vi "ke37xx Configure Filter.vi"(0 "VISA Resource Name":refnum<visa-resource-name>, 5 "Enabled (False)":bool, 7 "Filter Count (1)":u8=1 min=1 max=100, 9 "Filter Type (0: Repeating Average)":enum16{"Repeating Average", "Moving Average"}(ring), 11 "error in (no error)":errorcluster, 12 "Window (0.1)":dbl=0.1 min=0.0 max=10.0) -> (4 "VISA Resource Name Out":refnum<visa-resource-name>, 15 "error out":errorcluster)   [LabVIEW 2009, in "Keithley 3700 Series.lvlib"]
doc: "This VI allows you to configure the measurement filter."
uses:
  <instrlib>/Keithley 3706/Keithley 3700 Series.lvlib
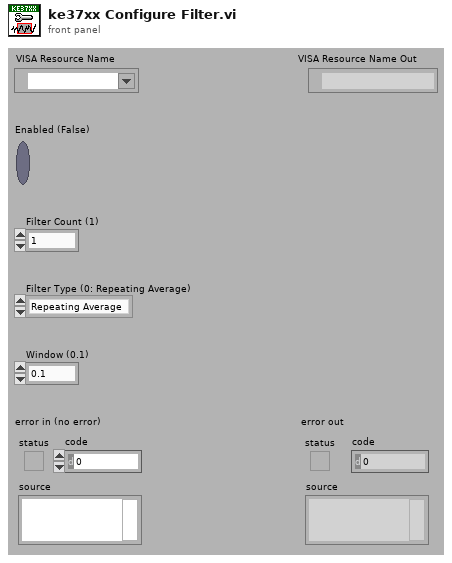
[diagram p1: front panel]
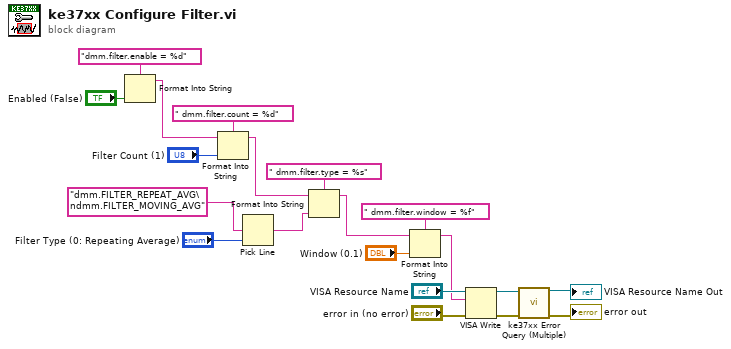
[diagram p0: block diagram]
diagram:
  n1 = Format Into String(format string="dmm.filter.enable = %d", "Enabled (False)") -> (resulting string=w8:string)  [unwired: 2 in, 1 out]
  n2 = Format Into String(format string=" dmm.filter.count = %d", initial string=w8, "Filter Count (1)") -> (resulting string=w7:string)  [unwired: 1 in, 1 out]
  n3 = Pick Line(multi-line string="dmm.FILTER_REPEAT_AVG\ndmm.FILTER_MOVING_AVG", line index="Filter Type (0: Repeating Average)") -> (output string=w2:string)  [unwired: 1 out]
  n4 = Format Into String(format string=" dmm.filter.type = %s", initial string=w7, w2) -> (resulting string=w6:string)  [unwired: 1 in, 1 out]
  n5 = Format Into String(format string=" dmm.filter.window = %f", initial string=w6, "Window (0.1)") -> (resulting string=w1:string)  [unwired: 1 in, 1 out]
  n6 = VISA Write(VISA resource name="VISA Resource Name", write buffer=w1, error in (no error)="error in (no error)") -> (VISA resource name out=w15:refnum<visa-resource-name>, error out=w14:errorcluster)  [unwired: 1 out]
  n7 = call <instrlib>:"ke37xx Error Query (Multiple).vi"("VISA resource name"=w15, "error in (no error)"=w14) -> ("VISA resource name out"=→"VISA Resource Name Out":refnum<visa-resource-name>, "error out"=→"error out":errorcluster)  [unwired: 12 out]
